vi "VI Tree.vi"   [LabVIEW 2012, in "Phidget Pressure Sensor.lvlib"]
doc: "${PressureSensor:VITreeHeader}"
uses:
  <instrlib>/Phidgets/Phidget Pressure Sensor/Phidget Pressure Sensor.lvlib
  <instrlib>/Phidgets/Phidget Pressure Sensor/Public/PressureSensorStart.vi
  <instrlib>/Phidgets/Phidget Pressure Sensor/Public/PressureSensorOpen.vi
  <instrlib>/Phidgets/Phidget Pressure Sensor/Public/PressureSensorClose.vi
panel:
  # "(c) 2015 Phidgets Inc..  ALL RIGHTS RESERVED."
  # "SEE DIAGRAM\nFOR VI TREE."
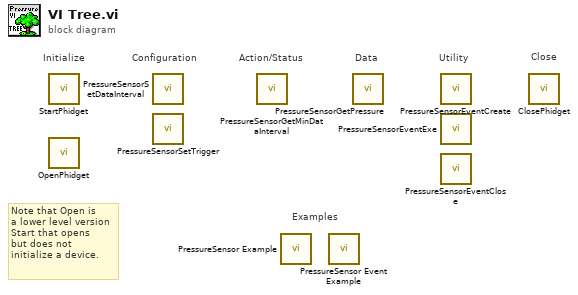
[diagram p0: block diagram]
diagram:
  # "Note that Open is\na lower level version\nStart that opens\nbut does not \ninitialize a device."
  # "Examples"
  # "Configuration"
  # "Utility"
  # "Data"
  # "Action/Status"
  # "Close"
  # "Initialize"
  n1 = call-poly <instrlib>:"StartPhidget.vi"() -> ()  [unwired: 12 in, 4 out]
  n2 = call-poly <instrlib>:"OpenPhidget.vi"() -> ()  [unwired: 8 in, 4 out]
  n3 = call <instrlib>:"PressureSensorSetDataInterval.vi"() -> ()  [unwired: 9 in, 2 out]
  n4 = call <instrlib>:"PressureSensorSetTrigger.vi"() -> ()  [unwired: 9 in, 2 out]
  n5 = call <instrlib>:"PressureSensorGetMinDataInterval.vi"() -> ()  [unwired: 8 in, 3 out]
  n6 = call <instrlib>:"PressureSensor Example.vi"() -> ()  [unwired: 12 in]
  n7 = call <instrlib>:"PressureSensor Event Example.vi"() -> ()  [unwired: 12 in]
  n8 = call <instrlib>:"PressureSensorGetPressure.vi"() -> ()  [unwired: 8 in, 3 out]
  n9 = call <instrlib>:"PressureSensorEventCreate.vi"() -> ()  [unwired: 9 in, 3 out]
  n10 = call <instrlib>:"PressureSensorEventExe.vi"() -> ()  [unwired: 5 in, 7 out]
  n11 = call <instrlib>:"PressureSensorEventClose.vi"() -> ()  [unwired: 10 in, 2 out]
  n12 = call-poly <instrlib>:"ClosePhidget.vi"() -> ()  [unwired: 11 in, 1 out]
